vi "Particle Classification.vi"() -> ()   [LabVIEW 2014]
doc: "This example shows how to use the classification VIs in NI Vision.\n\nClassification quickly identifies and classifies unknown objects in inspection images. First, use the Classification Training Interface to teach your application the types, or classes, of objects you want to classify. The Classification Training Interface creates a classifier file, which you then use to classify unknown objects into one of the classes you trained."
uses:
  <vilib>/vision/NI_Vision_Development_Module.lvlib
panel:
  out "Image":T1(plugin-control)
  # "Overview: Demonstrates how to use the IMAQ Classify function with a binary classifier file to dynamically find the bounding box of the particles and classify them.\nRequirements: Vision Development Software.\nInstructions: Run the VI."
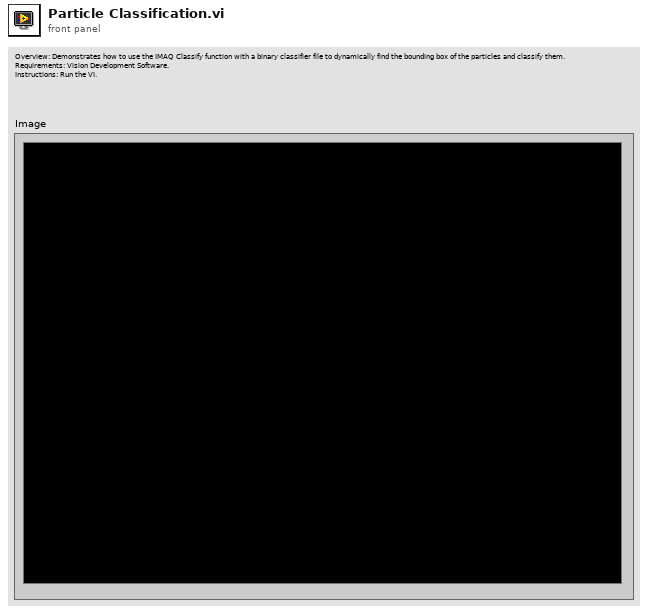
[diagram p1: front panel]
types:
  T1 = typedef "IMAQ Image.ctl" = refnum<image>
  T2 = typedef "IMAQ Classifier Session.ctl" = refnum<k1>
  T3 = typedef "ROI Descriptor" = cluster{"Global Rectangle":i32[], "Contours":cluster{"ID":enum32{"External", "Internal"}, "Type":u32, "Coordinates":i32[]}[]}
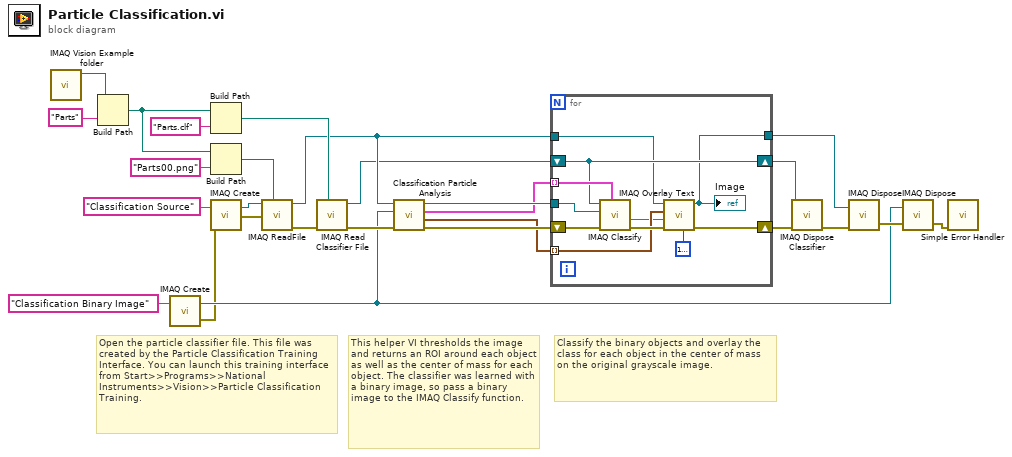
[diagram p0: block diagram]
diagram:
  # "Open the particle classifier file. This file was created by the Particle Classification Training Interface. You can launch this training interface from Start>>Programs>>National Instruments>>Vision>>Particle Classification Training."
  # "Classify the binary objects and overlay the class for each object in the center of mass on the original grayscale image."
  # "This helper VI thresholds the image and returns an ROI around each object as well as the center of mass for each object. The classifier was learned with a binary image, so pass a binary image to the IMAQ Classify function."
  n1 = call "IMAQ Vision Example folder.vi"() -> ("Example Image Path"=w20:path)  [unwired: 11 in]
  n2 = Build Path(base path=w20, name or relative path="Parts") -> (appended path=w18:path)
  n3 = call "IMAQ Create"("Image Name"="Classification Binary Image") -> ("New Image"=w6:T1, "error out"=w4:errorcluster)  [unwired: 3 in, 1 out]
  n4 = Build Path(base path=w18, name or relative path="Parts.clf") -> (appended path=w17:path)
  n5 = Build Path(base path=w18, name or relative path="Parts00.png") -> (appended path=w15:path)
  n6 = call "IMAQ Create"("Image Name"="Classification Source", "error in (no error)"=w4) -> ("New Image"=w14:T1, "error out"=w13:errorcluster)  [unwired: 2 in, 1 out]
  n7 = call "IMAQ ReadFile"("File Path"=w15, "error in (no error)"=w13, "Image"=w14) -> ("error out"=w16:errorcluster, "Image Out"=w5:T1)  [unwired: 4 in, 3 out]
  n8 = call "IMAQ Read Classifier File"("File Path"=w17, "error in (no error)"=w16) -> ("error out"=w11:errorcluster, "Classifier Session"=w1:T2)  [unwired: 2 in, 6 out]
  n9 = call "Classification Particle Analysis.vi"("error in (no error)"=w11, "Image Dest"=w6, "Image Source"=w5) -> ("error out"=w26:errorcluster, "Center of Masses"=w25:cluster{"X":dbl, "Y":dbl}[], "ROIs"=w24:T3[], "Image Out"=w27:T1)  [unwired: 5 in]
  n10 = for {
    tunnel: w24 -> [w37] mode=indexing
    tunnel: w25 -> [w33] mode=indexing
    tunnel: w27 -> [w36]
    shift-right: [w35] -> w10
    shift-left: w1 -> [w35]
    shift-right: [w31] -> w9
    shift-left: w26 -> [w38]
    tunnel: w5 -> [w29]
    tunnel: [w28] -> w3
    n11 = call "IMAQ Classify"("ROI Descriptor"=w37, "error in (no error)"=w38, "Image"=w36, "Classifier Session"=w35) -> ("error out"=w34:errorcluster, "Class"=w32:string)  [unwired: 6 out]
    n12 = call "IMAQ Overlay Text"("BG Color (Transparent)"=u32 16777226, "error in (no error)"=w34, "String"=w32, "Origin"=w33, "Image"=w29) -> ("error out"=w31:errorcluster, "Image Out"=w28:T1)  [unwired: 5 in]
    "Image" <- w28
  }
  n13 = call "IMAQ Dispose Classifier"("error in (no error)"=w9, "Classifier Session"=w10) -> ("error out"=w8:errorcluster)  [unwired: 9 out]
  n14 = call "IMAQ Dispose"("Image"=w3, "error in (no error)"=w8) -> ("error out"=w7:errorcluster)  [unwired: 1 in, 3 out]
  n15 = call "IMAQ Dispose"("Image"=w6, "error in (no error)"=w7) -> ("error out"=w2:errorcluster)  [unwired: 1 in, 3 out]
  n16 = call <vilib>:"Simple Error Handler.vi"("error in (no error)"=w2) -> ()  [unwired: 4 in, 5 out]
